vi "Get T -- LS340.vi"(6 "sensor":i32=1, 7 "GPIB Adress":i16, 8 "error in (no error)":errorcluster) -> (0 "error out":errorcluster, 2 "sensor data string":string, 3 "sensor Temperature":dbl format="%.3f")   [LabVIEW 2015]
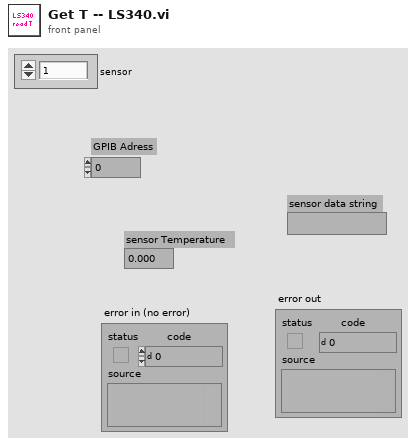
[diagram p1: front panel]
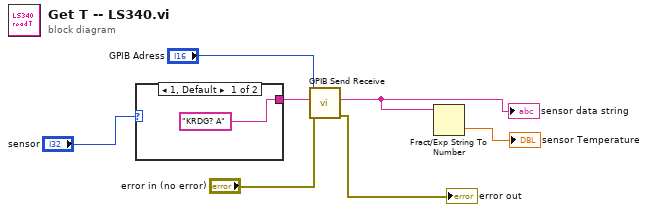
[diagram p0: block diagram]
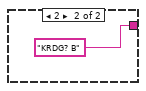
[diagram p2: hidden frame]
diagram:
  n1 = case shown="1, Default" "sensor" {
    tunnel: ["KRDG? A" ("data string") "KRDG? B" ("data string")] -> w7
    frame 1, Default {
    }
    frame 2 {
    }
  }
  n2 = call "GPIB Send Receive.vi"("error in (no error)"="error in (no error)", "data string in"=w7, "GPIB Adress"="GPIB Adress") -> ("error out"=→"error out":errorcluster, "data string out"=w5:string)  [unwired: 6 in, 1 out]
  "sensor data string" <- w5
  n3 = Fract/Exp String To Number(string=w5) -> (number=→"sensor Temperature":dbl)  [unwired: 3 in, 1 out]
